vi "ex7-11.vi"() -> ()   [LabVIEW 2013]
panel:
  out "output array":dbl[](array[numeric])
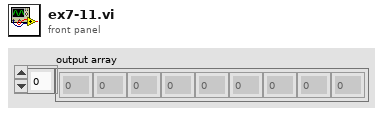
[diagram p1: front panel]
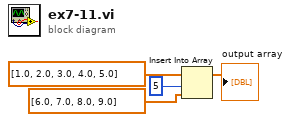
[diagram p0: block diagram]
diagram:
  n1 = Insert Into Array(array=dbl[] [1.0, 2.0, 3.0, 4.0, 5.0], index=5, new element=dbl[] [6.0, 7.0, 8.0, 9.0] ("array")) -> (→"output array":dbl[])
